vi "18.5 Color Classification.vi"() -> ()   [LabVIEW 2017]
doc: "This example shows how to use the classification VIs in NI Vision.\n\nClassification quickly identifies and classifies unknown objects in inspection images. First, use the Classification Training Interface to teach your application the types, or classes, of objects you want to classify. The Classification Training Interface creates a classifier file, which you then use to classify unknown objects into one of the classes you trained."
uses:
  <vilib>/vision/NI_Vision_Development_Module.lvlib
panel:
  out "Class":string
  out "Scores":T1 {"Identification Score" format="%.2f"; "Classification Score" format="%.2f"}
  in  "stop":bool
  out "Image":T2(plugin-control)
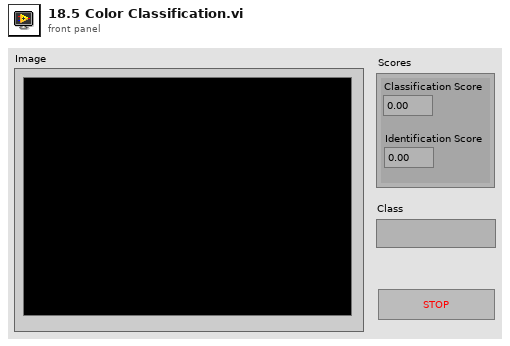
[diagram p1: front panel]
types:
  T1 = cluster{"Classification Score":sgl, "Identification Score":sgl}
  T2 = typedef "IMAQ Image.ctl" = refnum<image>
  T3 = typedef "Image Type" = u32
  T4 = typedef "IMAQ Rectangle" = cluster{"Left":i32, "Top":i32, "Right":i32, "Bottom":i32, "Rotation":dbl}
  T5 = typedef "IMAQ Classifier Session.ctl" = refnum<k1>
  T6 = typedef "ROI Descriptor" = cluster{"Global Rectangle":i32[], "Contours":cluster{"ID":enum32{"External", "Internal"}, "Type":u32, "Coordinates":i32[]}[]}
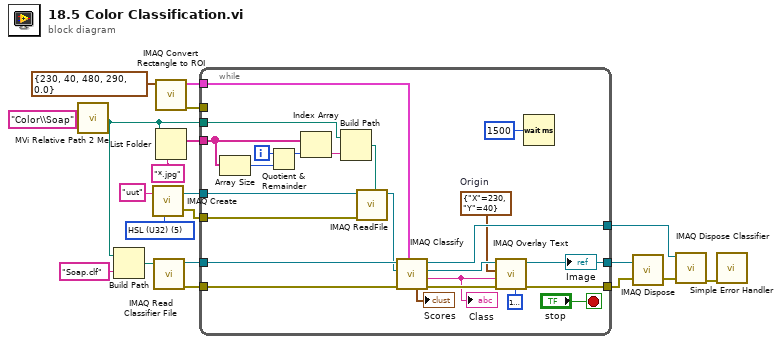
[diagram p0: block diagram]
diagram:
  w1 = T3 5 items=["Grayscale (U8)", "Grayscale (I16)", "Grayscale (SGL)", "Complex (CSG)", "RGB (U32)", "HSL (U32)", "RGB (U64)", "Grayscale (U16)"] ("Image Type")
  n1 = call "MVi Relative Path 2 Me.vi"("Relative Path"="Color\\Soap" ("name or relative path")) -> ("Appended Dir"=w9:path)  [unwired: 5 in, 1 out]
  n2 = Build Path(base path=w9, name or relative path="Soap.clf") -> (appended path=w18:path)
  n3 = call "IMAQ Create"("Image Name"="uut", "Image Type"=w1) -> ("New Image"=w11:T2, "error out"=w10:errorcluster)  [unwired: 2 in, 1 out]
  n4 = call "IMAQ Read Classifier File"("File Path"=w18) -> ("error out"=w14:errorcluster, "Classifier Session"=w17:T5)  [unwired: 3 in, 6 out]
  n5 = call "IMAQ Convert Rectangle to ROI"("Rectangle"=T4 {"Left"=230, "Top"=40, "Right"=480, "Bottom"=290, "Rotation"=0.0}) -> ("error out"=w7:errorcluster, "ROI Descriptor"=w8:T6)  [unwired: 8 in]
  n6 = List Folder(path=w9, pattern="*.jpg") -> (filenames=w12:string[])  [unwired: 2 in, 3 out]
  n7 = while {
    tunnel: [w44] -> w5
    tunnel: w17 -> [w43]
    tunnel: [w28] -> w15
    tunnel: w14 -> [w29]
    tunnel: w12 -> [w36]
    tunnel: w11 -> [w35]
    tunnel: w10 -> [w30]
    tunnel: w9 -> [w33]
    tunnel: w8 -> [w27]
    tunnel: w7 -> [_]
    tunnel: [w23] -> w2
    i -> [w37]
    stop <- "stop" stop-if-true
    w22 = cluster{"X":i32, "Y":i32} {"X"=230, "Y"=40}  # Origin
    n8 = Array Size(array=w36) -> (size(s)=w39:i32)
    n9 = Quotient & Remainder(x=w37, y=w39) -> (x-y*floor(x/y)=w38:i32)  [unwired: 1 out]
    n10 = Index Array(array=w36, index=w38) -> (element=w34:string)
    n11 = Build Path(base path=w33, name or relative path=w34) -> (appended path=w32:path)
    n12 = call "IMAQ ReadFile"("File Path"=w32, "error in (no error)"=w30, "Image"=w35) -> ("Image Out"=w31:T2)  [unwired: 4 in, 4 out]
    n13 = call "IMAQ Classify"("ROI Descriptor"=w27, "error in (no error)"=w29, "Image"=w31, "Classifier Session"=w43) -> ("error out"=w42:errorcluster, "Class"=w40:string, "Image (dup)"=w25:T2, "Classifier Session (dup)"=w23:T5, "Scores"=→"Scores":T1)  [unwired: 3 out]
    "Class" <- w40
    n14 = call "IMAQ Overlay Text"("BG Color (Transparent)"=u32 16777226, "error in (no error)"=w42, "String"=w40, "Origin"=w22, "Image"=w25) -> ("error out"=w44:errorcluster, "Image Out"=w28:T2)  [unwired: 5 in]
    "Image" <- w28
    n15 = Wait (ms)(milliseconds to wait=u32 1500) -> ()  [unwired: 1 out]
  }
  n16 = call "IMAQ Dispose"("Image"=w15, "error in (no error)"=w5) -> ("error out"=w4:errorcluster)  [unwired: 1 in, 3 out]
  n17 = call "IMAQ Dispose Classifier"("error in (no error)"=w4, "Classifier Session"=w2) -> ("error out"=w3:errorcluster)  [unwired: 9 out]
  n18 = call <vilib>:"Simple Error Handler.vi"("error in (no error)"=w3) -> ()  [unwired: 4 in, 5 out]
